vi "PowerOffCalibration.vi"(0 "Tasks In":T1, 5 "Offset Cali Steps":dbl=100.0, 11 "error in":errorcluster) -> (4 "Tasks Out":T1, 6 "V_DC Array":dbl[](array[numeric]), 8 "d13 Array":dbl[](array[numeric]), 10 "d24 Array":dbl[](array[numeric]), 15 "error out":errorcluster)   [LabVIEW 2018]
uses:
  <vilib>/DAQmx/read.llb/DAQmx Read (Analog 2D DBL NChan NSamp).vi
  <vilib>/DAQmx/read.llb/DAQmx Read (Analog 1D DBL 1Chan NSamp).vi
  <vilib>/DAQmx/miscellaneous.llb/DAQmx Fill In Error Info.vi
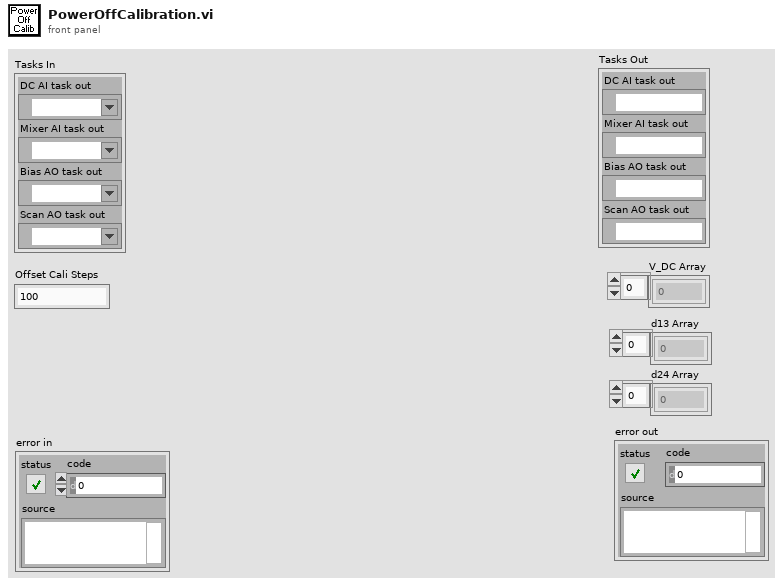
[diagram p1: front panel]
types:
  T1 = cluster{"DC AI task out":refnum<k21>, "Mixer AI task out":refnum<k21>, "Bias AO task out":refnum<k21>, "Scan AO task out":refnum<k21>}
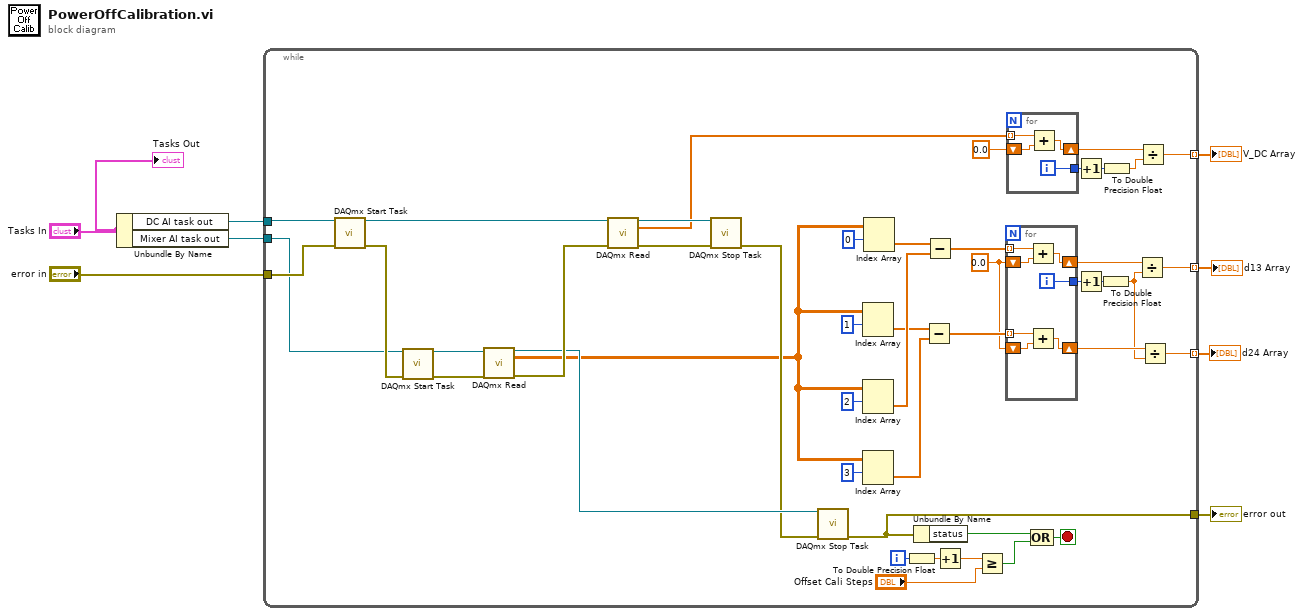
[diagram p0: block diagram]
diagram:
  n1 = Unbundle By Name("Tasks In") -> ("DC AI task out"=w6:refnum<k21>, "Mixer AI task out"=w5:refnum<k21>)
  n2 = while {
    tunnel: "error in" -> [w52]
    tunnel: [w31] -> w4
    tunnel: [w30] -> w3 mode=indexing
    tunnel: w6 -> [w28]
    tunnel: w5 -> [w29]
    tunnel: [w10] -> w2 mode=indexing
    tunnel: [w9] -> w1 mode=indexing
    i -> [w42]
    stop <- w43 stop-if-true
    w13 = 0.0
    n3 = call <vilib>:"DAQmx Start Task.vi"("task/channels in"=w28, "error in"=w52) -> ("task out"=w53:refnum<k21>, "error out"=w37:errorcluster)  [unwired: 12 in]
    n4 = call <vilib>:"DAQmx Start Task.vi"("task/channels in"=w29, "error in"=w37) -> ("task out"=w36:refnum<k21>, "error out"=w35:errorcluster)  [unwired: 12 in]
    n5 = call-poly <vilib>:"DAQmx Read.vi"("task/channels in"=w36, "error in"=w35) -> ("task out"=w33:refnum<k21>, "data"=w23:dbl[][], "error out"=w34:errorcluster)  [unwired: 11 in]
    n6 = call-poly <vilib>:"DAQmx Read.vi"("task/channels in"=w53, "error in"=w34) -> ("task out"=w54:refnum<k21>, "data"=w45:dbl[], "error out"=w51:errorcluster)  [unwired: 11 in]
    n7 = call <vilib>:"DAQmx Stop Task.vi"("task/channels in"=w54, "error in"=w51) -> ("error out"=w32:errorcluster)  [unwired: 12 in, 1 out]
    n8 = call <vilib>:"DAQmx Stop Task.vi"("task/channels in"=w33, "error in"=w32) -> ("error out"=w31:errorcluster)  [unwired: 12 in, 1 out]
    n9 = Index Array(array=w23, index (row)=1) -> (element=w20:dbl[])  [unwired: 1 in]
    n10 = Index Array(array=w23, index (row)=2) -> (element=w21:dbl[])  [unwired: 1 in]
    n11 = Index Array(array=w23, index (row)=3) -> (element=w19:dbl[])  [unwired: 1 in]
    n12 = Index Array(array=w23, index (row)=0) -> (element=w22:dbl[])  [unwired: 1 in]
    n13 = To Double Precision Float(number=w42) -> (double precision float=w41:dbl)
    n14 = Unbundle By Name(w31) -> ("status"=w44:bool)
    n15 = Subtract(x=w20, y=w19) -> (x-y=w14:dbl[])
    n16 = Subtract(x=w22, y=w21) -> (x-y=w15:dbl[])
    n17 = Increment(x=w41) -> (x+1=w40:dbl)
    n18 = Greater Or Equal?(x=w40, y="Offset Cali Steps") -> (x >= y?=w39:bool)
    n19 = for {
      tunnel: w15 -> [w61] mode=indexing
      shift-right: [w59] -> w18
      shift-left: w13 -> [w60]
      tunnel: [w58] -> w16
      tunnel: w14 -> [w57] mode=indexing
      shift-right: [w55] -> w12
      shift-left: w13 -> [w56]
      i -> [w58]
      n20 = Add(x=w61, y=w60) -> (x+y=w59:dbl)
      n21 = Add(x=w57, y=w56) -> (x+y=w55:dbl)
    }
    n22 = for {
      tunnel: w45 -> [w65] mode=indexing
      shift-right: [w63] -> w46
      shift-left: 0.0 -> [w64]
      tunnel: [w62] -> w48
      i -> [w62]
      n23 = Add(x=w65, y=w64) -> (x+y=w63:dbl)
    }
    n24 = Compound Arithmetic op=OR(w44, w39) -> (w43:bool)
    n25 = Increment(x=w48) -> (x+1=w47:i32)
    n26 = Increment(x=w16) -> (x+1=w17:i32)
    n27 = To Double Precision Float(number=w17) -> (double precision float=w11:dbl)
    n28 = To Double Precision Float(number=w47) -> (double precision float=w49:dbl)
    n29 = Divide(x=w18, y=w11) -> (x/y=w10:dbl)
    n30 = Divide(x=w46, y=w49) -> (x/y=w30:dbl)
    n31 = Divide(x=w12, y=w11) -> (x/y=w9:dbl)
  }
  "error out" <- w4
  "V_DC Array" <- w3
  "d13 Array" <- w2
  "d24 Array" <- w1
  "Tasks Out" <- "Tasks In"
